vi "LVITX IBW aperture Commands.vi"(1 "input string":string="Display 'y_#wave#' vs 'x_#wave#'\nAppendToGraph 'y_#wave#' vs 'x_#wave#'\nLabel bottom \"#labelX#\"\nLabel left \"#labelY#\"\nModifyGraph rgb('y_#wave#')=(#r#,#g#,#b#)\nLegend/C/N=text0", 2 "Y label":string, 3 "X label":string, 4 "wavenames":string[](array[string])=["TEST1.5.Vx", "TEST1.5.Vy"]) -> (0 "result string":string="Display 'y_TEST1.5.Vx' vs 'x_TEST1.5.Vx'\nAppendToGraph 'y_TEST1.5.Vy' vs 'x_TEST1.5.Vy'\nLabel bottom \"bias (V)\"\nLabel left \"energyy (eV)\"\nModifyGraph rgb('y_TEST1.5.Vx')=(65280,0,0)\nModifyGraph rgb('y_TEST1.5.Vy')=(0,65280,45568)\nLegend/C/N=text0/J/X=-30.00/Y=40.00")   [LabVIEW 2013]
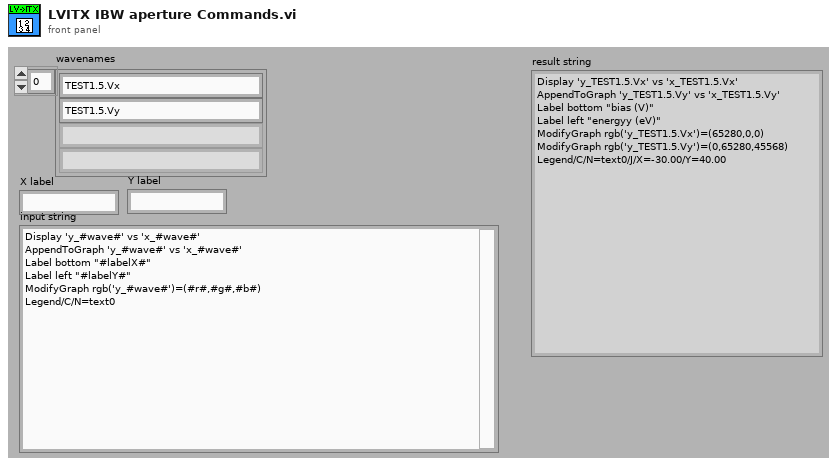
[diagram p1: front panel]
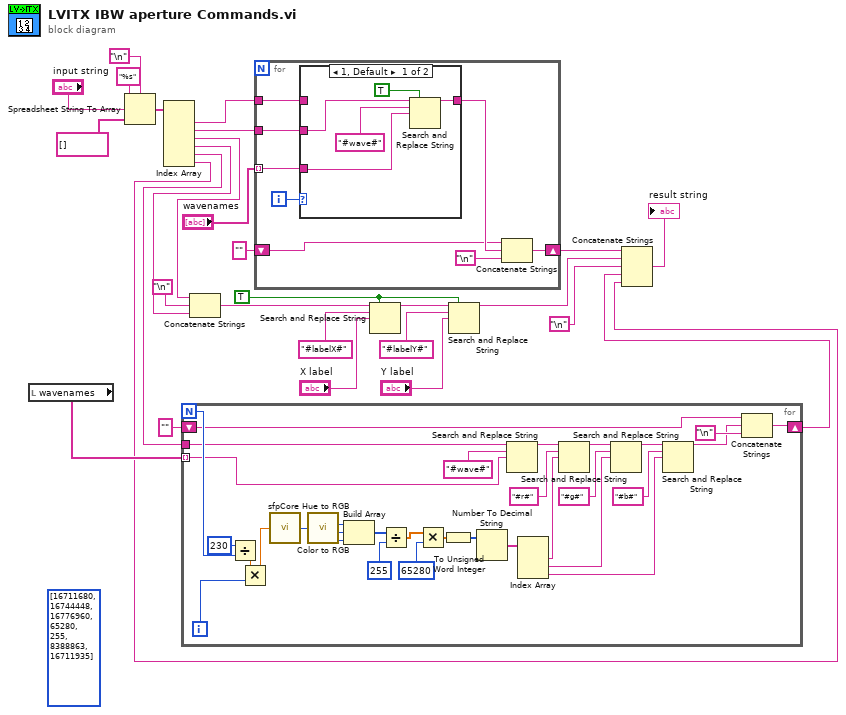
[diagram p0: block diagram]
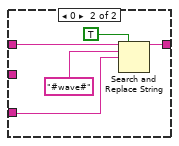
[diagram p2: hidden frame]
diagram:
  w7 = TRUE ("replace all? (F)")
  (unwired) u32[] [16711680, 16744448, 16776960, 65280, 255, 8388863, 16711935]
  n1 = local read "wavenames"() -> (w5:string[])
  n2 = Spreadsheet String To Array(delimiter (Tab)="\n", format string="%s", spreadsheet string="input string", array type (2D Dbl)=string[] []) -> (array=w19:string[])
  n3 = Index Array(array=w19) -> (element #1=w18:string, element #2=w17:string, element #3=w14:string, element #4=w12:string, element #5=w8:string, element #6=w2:string)  [unwired: 6 in]
  n4 = for {
    N -> [w49]
    tunnel: w8 -> [w44]
    tunnel: w5 -> [w37] mode=indexing
    shift-right: [w40] -> w1
    shift-left: "" -> [w39]
    i -> [w48]
    n5 = Divide(x=230, y=w49) -> (x/y=w51:dbl)
    n6 = Multiply(x=w51, y=w48) -> (x*y=w47:dbl)
    n7 = call <userlib>:"sfpCore Hue to RGB.vi"("hue value"=w47) -> ("output color"=w53:u32)
    n8 = call <vilib>:"Color to RGB.vi"("Color"=w53) -> ("R"=w58:u8, "G"=w59:u8, "B"=w60:u8)  [unwired: 1 out]
    n9 = Build Array(w58, w59, w60) -> (w57:u8[])
    n10 = Divide(x=w57, y=255) -> (x/y=w52:dbl[])
    n11 = Multiply(x=w52, y=65280) -> (x*y=w54:dbl[])
    n12 = To Unsigned Word Integer(number=w54) -> (unsigned 16bit integer=w46:u16[])
    n13 = Number To Decimal String(number=w46) -> (decimal integer string=w32:string[])  [unwired: 1 out]
    n14 = Search and Replace String(input string=w44, search string="#wave#", replace string=w37) -> (result string=w45:string)  [unwired: 1 in, 7 out]
    n15 = Index Array(array=w32) -> (element #1=w31:string, element #2=w30:string, element #3=w29:string)  [unwired: 3 in]
    n16 = Search and Replace String(input string=w45, search string="#r#", replace string=w31) -> (result string=w43:string)  [unwired: 1 in, 7 out]
    n17 = Search and Replace String(input string=w43, search string="#g#", replace string=w30) -> (result string=w42:string)  [unwired: 1 in, 7 out]
    n18 = Search and Replace String(input string=w42, search string="#b#", replace string=w29) -> (result string=w36:string)  [unwired: 1 in, 7 out]
    n19 = Concatenate Strings(w39, w36, "\n") -> (w40:string)
  }
  n20 = Concatenate Strings(w14, "\n", w12) -> (w15:string)
  n21 = for {
    tunnel: "wavenames" -> [w66] mode=indexing
    tunnel: w18 -> [w68]
    tunnel: w17 -> [w67]
    shift-right: [w64] -> w23
    shift-left: "" -> [w61]
    i -> [w65]
    n22 = case shown="1, Default" w65 {
      tunnel: w68 -> [_ w76]
      tunnel: w67 -> [w71 _]
      tunnel: w66 -> [w72 w77]
      tunnel: [w70 w75] -> w63
      frame 1, Default {
        n23 = Search and Replace String(replace all?=TRUE ("replace all? (F)"), input string=w71, search string="#wave#", replace string=w72) -> (result string=w70:string)  [unwired: 1 in, 6 out]
      }
      frame 0 {
        n24 = Search and Replace String(replace all?=TRUE ("replace all? (F)"), input string=w76, search string="#wave#", replace string=w77) -> (result string=w75:string)  [unwired: 1 in, 6 out]
      }
    }
    n25 = Concatenate Strings(w61, w63, "\n") -> (w64:string)
  }
  n26 = Search and Replace String(replace all?=w7, input string=w15, search string="#labelX#", replace string="X label") -> (result string=w11:string)  [unwired: 1 in, 6 out]
  n27 = Search and Replace String(replace all?=w7, input string=w11, search string="#labelY#", replace string="Y label") -> (result string=w4:string)  [unwired: 1 in, 6 out]
  n28 = Concatenate Strings(w23, w4, "\n", w1, w2) -> (→"result string":string)
